vi "Turbine Optimizer.vi"() -> ()   [LabVIEW 2021]
panel:
  in  "Flow (mB/t)":dbl
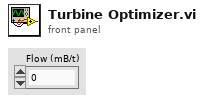
[diagram p1: front panel]
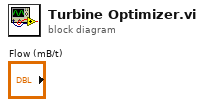
[diagram p0: block diagram]
diagram:
